vi "FormatEnum.vi"(1 "enum":variant) -> (0 "value":string)   [LabVIEW 2014, in "Raspberry Pi Compatible Compiler for LabVIEW.lvlib" / "PythonConfiguration.lvclass"]
uses:
  PythonConfiguration.lvclass
  <vilib>/Utility/VariantDataType/VariantType.lvlib
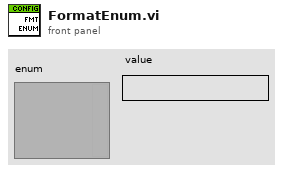
[diagram p1: front panel]
types:
  T1 = typedef "VariantType.lvlib/Type.ctl" = enum8{"Invalid Type", "Void", "I8", "I16", "I32", "I64", "U8", "U16", "U32", "U64", "Single Float", "Double Float", "Extended Float", "Single Complex", "Double Complex", "Extended Complex", "Enum U8", "Enum U16", "Enum U32", "Enum U64", "Single Float With Unit", "Double Float With Unit", "Extended Float With Unit", "Single Complex with Unit", "Double Complex with Unit", "Extended Complex with Unit", "Boolean", "String", "Path", "Picture", "Tag", "Array", "Cluster", "Variant", "LV Variant", "Waveform", "Timestamp", "Digital Waveform", "Digital Data", "ExpressData", "Refnum", "External Data", "VI", "Poly VI", "LabVIEW Class Instance", "Fixed Point"}
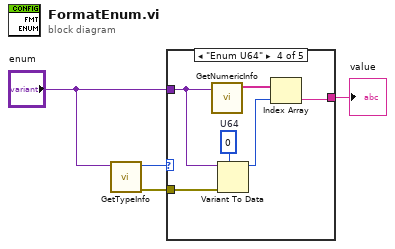
[diagram p0: block diagram]
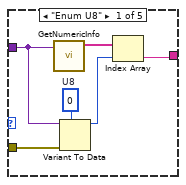
[diagram p2: hidden frame]
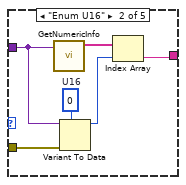
[diagram p3: hidden frame]
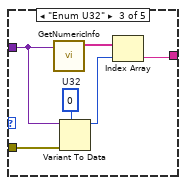
[diagram p4: hidden frame]
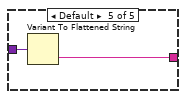
[diagram p5: hidden frame]
diagram:
  n1 = call <vilib>:"GetTypeInfo.vi"("Variant"="enum") -> ("error out"=w1:errorcluster, "Type Enum"=w2:T1)  [unwired: 6 in, 3 out]
  n2 = case shown="\"Enum U64\"" w2 {
    tunnel: [w5 w11 w17 w23 w30] -> w4
    tunnel: "enum" -> [w10 w16 w22 w28 w29]
    tunnel: w1 -> [w9 w15 w21 w27 _]
    frame "Enum U8" {
      w8 = u8 0  # U8
      n3 = call <vilib>:"GetNumericInfo.vi"("Variant"=w10) -> ("EnumNames"=w7:string[])  [unwired: 7 in, 3 out]
      n4 = Variant To Data(error in=w9, type=w8, Variant=w10) -> (data=w6:u8)  [unwired: 1 out]
      n5 = Index Array(array=w7, index=w6) -> (element=w5:string)
    }
    frame "Enum U16" {
      w14 = u16 0  # U16
      n6 = call <vilib>:"GetNumericInfo.vi"("Variant"=w16) -> ("EnumNames"=w13:string[])  [unwired: 7 in, 3 out]
      n7 = Variant To Data(error in=w15, type=w14, Variant=w16) -> (data=w12:u16)  [unwired: 1 out]
      n8 = Index Array(array=w13, index=w12) -> (element=w11:string)
    }
    frame "Enum U32" {
      w20 = u32 0  # U32
      n9 = call <vilib>:"GetNumericInfo.vi"("Variant"=w22) -> ("EnumNames"=w19:string[])  [unwired: 7 in, 3 out]
      n10 = Variant To Data(error in=w21, type=w20, Variant=w22) -> (data=w18:u32)  [unwired: 1 out]
      n11 = Index Array(array=w19, index=w18) -> (element=w17:string)
    }
    frame "Enum U64" {
      w26 = u64 0  # U64
      n12 = call <vilib>:"GetNumericInfo.vi"("Variant"=w28) -> ("EnumNames"=w25:string[])  [unwired: 7 in, 3 out]
      n13 = Variant To Data(error in=w27, type=w26, Variant=w28) -> (data=w24:u64)  [unwired: 1 out]
      n14 = Index Array(array=w25, index=w24) -> (element=w23:string)
    }
    frame Default {
      n15 = Variant To Flattened String(Variant=w29) -> (data string=w30:string)  [unwired: 1 out]
    }
  }
  "value" <- w4
